vi "ZoneVacuumCtrlBothSiHB.vi"(6 "Switches":T1, 7 "DecimalIn":u8, 8 "Error In":errorcluster, 9 "Position":enum16{"1", "2"}(ring), 10 "Zone":enum16{"ZoneA", "ZoneB", "ZoneC", "ZoneD"}(ring), 11 "ControlType":T2(ring)=enum."DecimalSwitch") -> (0 "Error Out":errorcluster, 2 "DecimalOut":u32, 3 "DecimalExpected":u32)   [LabVIEW 2021]
panel:
  out "Micro2 EM":bool
  out "Micro1":bool
  out "BP2":bool
  out "Si2":bool
  out "GHTool":bool
  out "GHPlate":bool
  out "BP1":bool
  out "Si1":bool
  out "HB1":bool
  out "PUT1":bool
  out "PUT2":bool
  out "HB2":bool
  # "Zone control"
  # "ZoneA Indicator"
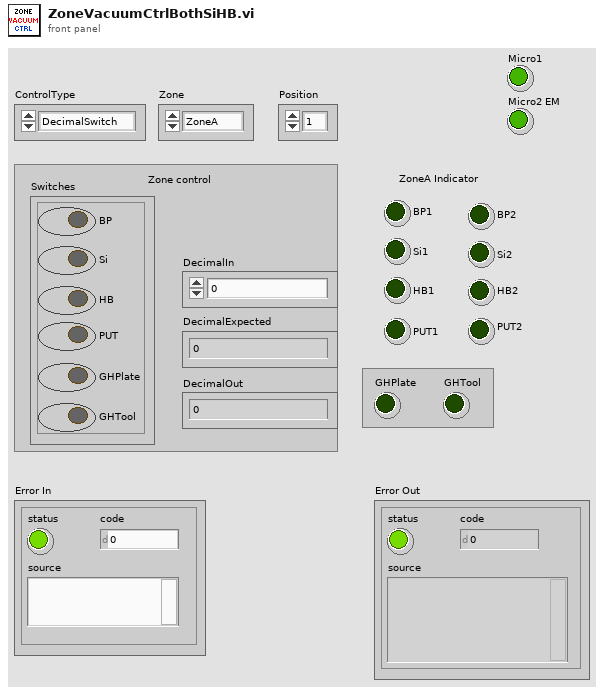
[diagram p1: front panel]
types:
  T1 = cluster{"BP":bool, "Si":bool, "HB":bool, "PUT":bool, "GHPlate":bool, "GHTool":bool}
  T2 = enum16{"BinarySwitch", "DecimalSwitch", "Conversion"}
  T3 = cluster{"data[0]":bool, "data[1]":bool, "data[2]":bool, "data[3]":bool, "data[4]":bool, "data[5]":bool, "data[6]":bool, "data[7]":bool, "data[8]":bool}
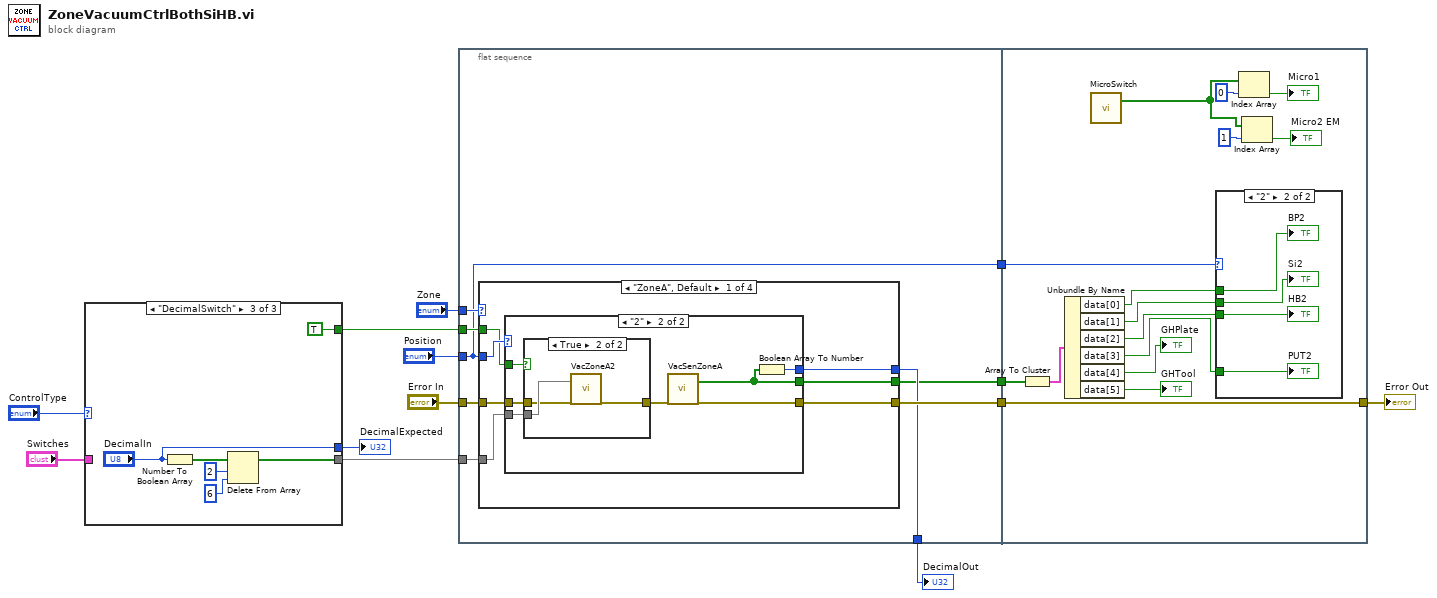
[diagram p0: block diagram]
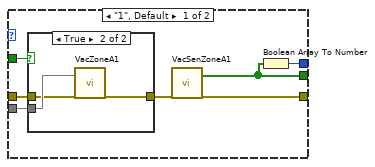
[diagram p2: hidden frame]
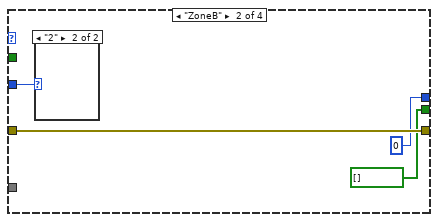
[diagram p5: hidden frame]
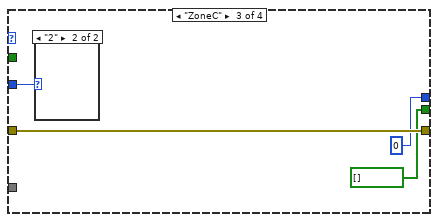
[diagram p7: hidden frame]
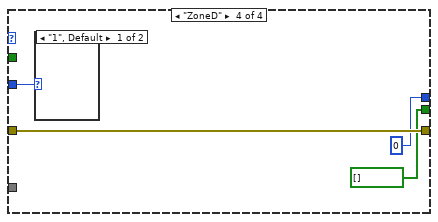
[diagram p9: hidden frame]
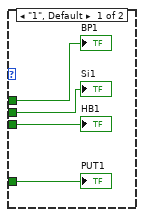
[diagram p11: hidden frame]
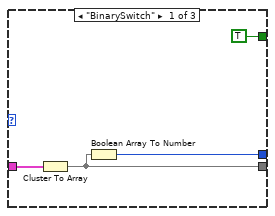
[diagram p12: hidden frame]
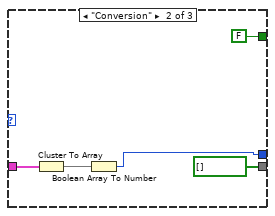
[diagram p13: hidden frame]
diagram:
  n1 = case shown="\"DecimalSwitch\"" "ControlType" {
    tunnel: [w16 bool[] [] ("Boolean array") w25] -> w11
    tunnel: [TRUE FALSE TRUE] -> w8
    tunnel: [w15 w20 "DecimalIn"] -> w7
    tunnel: "Switches" -> [w14 w18 _]
    frame "BinarySwitch" {
      n2 = Cluster To Array(cluster=w14) -> (array=w16:bool[])
      n3 = Boolean Array To Number(Boolean array=w16) -> (number=w15:u32)
    }
    frame "Conversion" {
      n4 = Cluster To Array(cluster=w18) -> (array=w19:bool[])
      n5 = Boolean Array To Number(Boolean array=w19) -> (number=w20:u32)
    }
    frame "DecimalSwitch" {
      n6 = Number To Boolean Array(number="DecimalIn") -> (Boolean array=w26:bool[])
      n7 = Delete From Array(array=w26, length=2, index=6) -> (array with subset deleted=w25:bool[])  [unwired: 1 out]
    }
  }
  "DecimalExpected" <- w7
  n8 = flat-sequence {
    tunnel: "Zone" -> [w36]
    tunnel: "Position" -> [w29]
    tunnel: w11 -> [w35]
    tunnel: "Error In" -> [w34]
    tunnel: w8 -> [w31]
    tunnel: [w33] -> w5
    tunnel: [w32] -> w4
    tunnel: [w30] -> w3
    tunnel: [w29] -> w1
    tunnel: w5 -> [w86]
    tunnel: w3 -> [w87]
    tunnel: [w86] -> w2
    tunnel: w1 -> [w83]
    frame #0 {
      n9 = case shown="\"ZoneA\", Default" w36 {
        tunnel: w29 -> [w43 w69 w73 w77]
        tunnel: w35 -> [w42 _ _ _]
        tunnel: w34 -> [w41 w68 w72 w76]
        tunnel: [w37 w68 w72 w76] -> w33
        tunnel: [w40 u32 0 u32 0 u32 0] -> w32
        tunnel: w31 -> [w39 _ _ _]
        tunnel: [w38 bool[] [] ("data") bool[] [] ("data") bool[] [] ("data")] -> w30
        frame "ZoneA", Default {
          n10 = case shown="\"2\"" w43 {
            tunnel: w42 -> [w50 w61]
            tunnel: w41 -> [w49 w56]
            tunnel: [w48 w58] -> w37
            tunnel: [w46 w60] -> w40
            tunnel: w39 -> [w45 w57]
            tunnel: [w44 w55] -> w38
            frame "1", Default {
              n11 = case shown="True" w45 {
                tunnel: w50 -> [_ w54]
                tunnel: w49 -> [w51 w53]
                tunnel: [w51 w52] -> w47
                frame False {
                }
                frame True {
                  n12 = call "VacZoneA1"("data"=w54, "error in"=w53) -> ("error out"=w52:errorcluster)  [unwired: 16 in, 1 out]
                }
              }
              n13 = call "VacSenZoneA1"("error in"=w47) -> ("data"=w44:bool[], "error out"=w48:errorcluster)  [unwired: 16 in, 1 out]
              n14 = Boolean Array To Number(Boolean array=w44) -> (number=w46:u32)
            }
            frame "2" {
              n15 = case shown="True" w57 {
                tunnel: w61 -> [_ w65]
                tunnel: [w62 w64] -> w59
                tunnel: w56 -> [w62 w63]
                frame False {
                }
                frame True {
                  n16 = call "VacZoneA2"("data"=w65, "error in"=w63) -> ("error out"=w64:errorcluster)  [unwired: 16 in, 1 out]
                }
              }
              n17 = call "VacSenZoneA"("error in"=w59) -> ("data"=w55:bool[], "error out"=w58:errorcluster)  [unwired: 16 in, 1 out]
              n18 = Boolean Array To Number(Boolean array=w55) -> (number=w60:u32)
            }
          }
        }
        frame "ZoneB" {
          n19 = case shown="\"2\"" w69 {
            frame "1", Default {
            }
            frame "2" {
            }
          }
        }
        frame "ZoneC" {
          n20 = case shown="\"2\"" w73 {
            frame "1", Default {
            }
            frame "2" {
            }
          }
        }
        frame "ZoneD" {
          n21 = case shown="\"1\", Default" w77 {
            frame "1", Default {
            }
            frame "2" {
            }
          }
        }
      }
    }
    frame #1 {
      n22 = Array To Cluster(array=w87) -> (cluster=w92:T3)
      n23 = Unbundle By Name(w92) -> ("data[0]"=w91:bool, "data[1]"=w90:bool, "data[2]"=w89:bool, "data[3]"=w88:bool, "data[4]"=→"GHPlate":bool, "data[5]"=→"GHTool":bool)
      n24 = call "MicroSwitch"() -> ("data"=w78:bool[])  [unwired: 17 in, 2 out]
      n25 = case shown="\"2\"" w83 {
        tunnel: w91 -> [w96 w100]
        tunnel: w90 -> [w95 w99]
        tunnel: w89 -> [w94 w98]
        tunnel: w88 -> [w93 w97]
        frame "1", Default {
          "PUT1" <- w93
          "HB1" <- w94
          "Si1" <- w95
          "BP1" <- w96
        }
        frame "2" {
          "BP2" <- w100
          "Si2" <- w99
          "HB2" <- w98
          "PUT2" <- w97
        }
      }
      n26 = Index Array(array=w78, index=0) -> (element=→"Micro1":bool)
      n27 = Index Array(array=w78, index=1) -> (element=→"Micro2 EM":bool)
    }
  }
  "Error Out" <- w2
  "DecimalOut" <- w4
